vi "Scanner_Tab_Data_To_Array.vi"(11 "Scanner Data":string) -> (3 "Array":string[](array[string]))   [LabVIEW 2017]
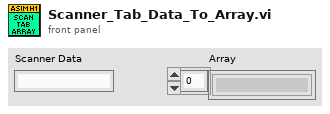
[diagram p1: front panel]
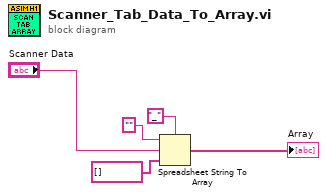
[diagram p0: block diagram]
diagram:
  n1 = Spreadsheet String To Array(delimiter (Tab)="_", format string="", spreadsheet string="Scanner Data", array type (2D Dbl)=string[] []) -> (array=→"Array":string[])
